vi "CreateOrAddLibrary.vi"   [LabVIEW 2017]
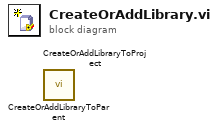
[diagram p0: block diagram]
diagram:
  n1 = call <vilib>:"CreateOrAddLibraryToParent.vi"() -> ()  [unwired: 9 in, 3 out]
  n2 = call <vilib>:"CreateOrAddLibraryToProject.vi"() -> ()  [unwired: 9 in, 3 out]
